vi "Flat sequential Structure.vi"() -> ()   [LabVIEW 2011]
panel:
  out "Z":dbl
  in  "Y":dbl
  in  "X":dbl
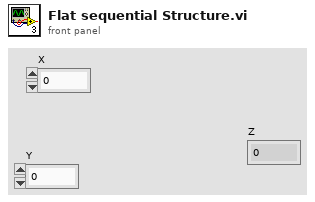
[diagram p1: front panel]
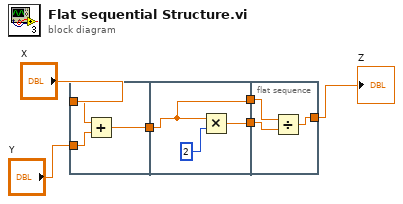
[diagram p0: block diagram]
diagram:
  n1 = flat-sequence {
    tunnel: "X" -> [w9]
    tunnel: "Y" -> [w8]
    tunnel: [w7] -> w4
    tunnel: w4 -> [w10]
    tunnel: [w11] -> w3
    tunnel: [w10] -> w2
    tunnel: w3 -> [w14]
    tunnel: w2 -> [w15]
    tunnel: [w13] -> w1
    frame #0 {
      n2 = Add(x=w9, y=w8) -> (x+y=w7:dbl)
    }
    frame #1 {
      n3 = Multiply(x=w10, y=2) -> (x*y=w11:dbl)
    }
    frame #2 {
      n4 = Divide(x=w15, y=w14) -> (x/y=w13:dbl)
    }
  }
  "Z" <- w1
